vi "fit_fix height and width.vi"() -> ()   [LabVIEW 2016] (continued)
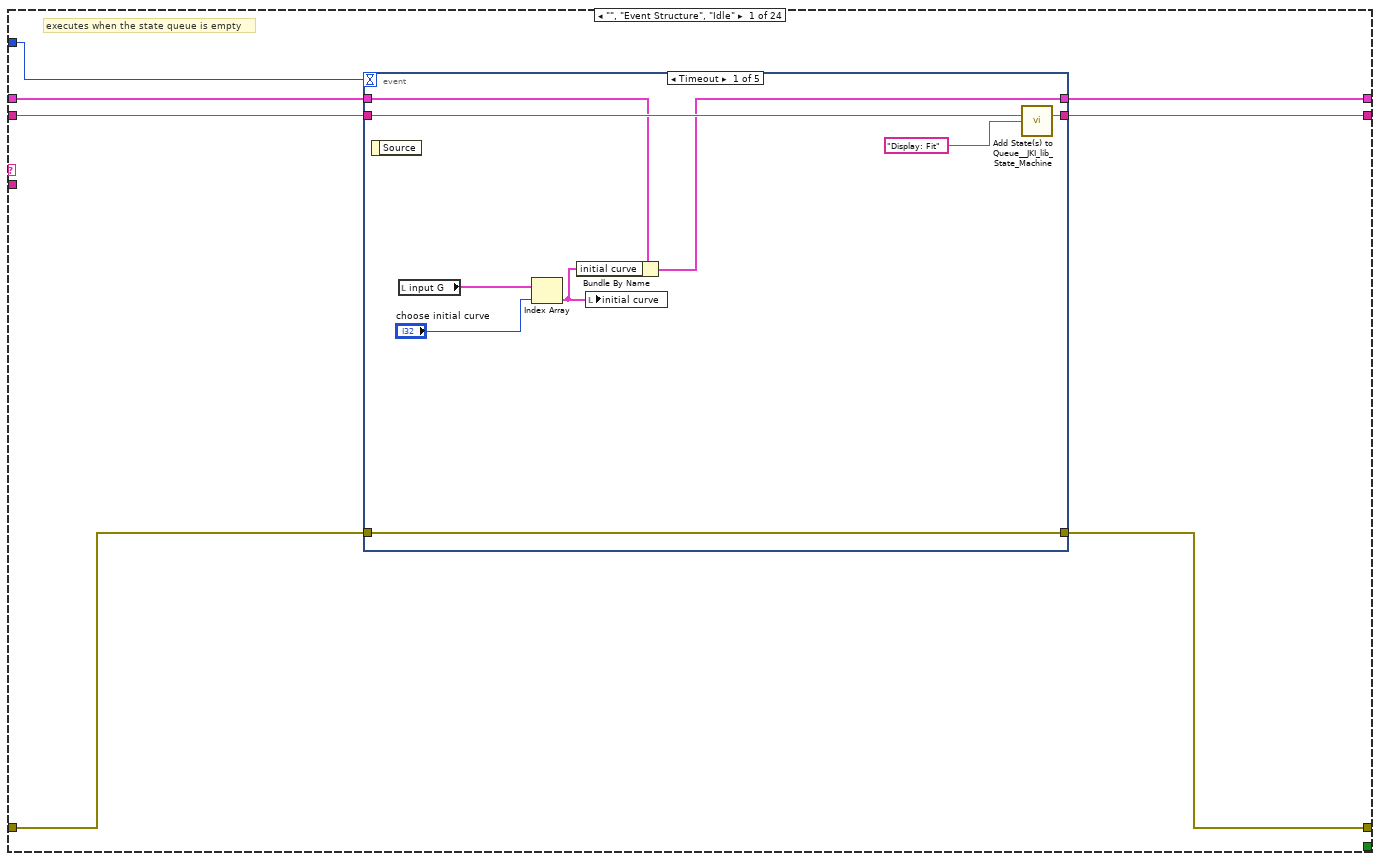
[diagram p3: hidden frame]
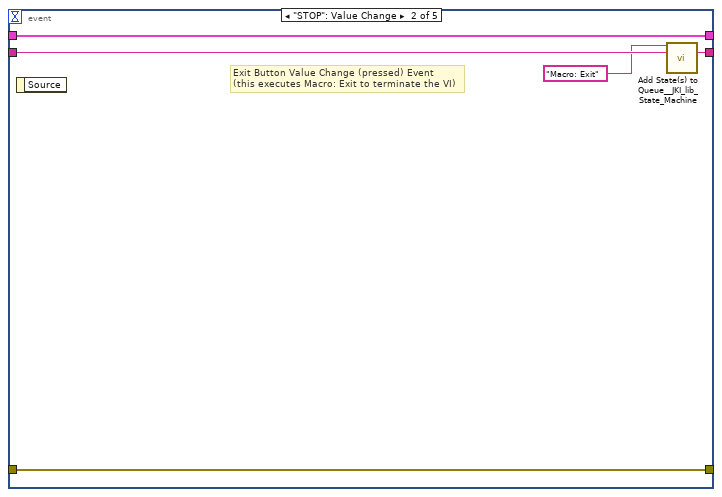
[diagram p4: hidden frame]
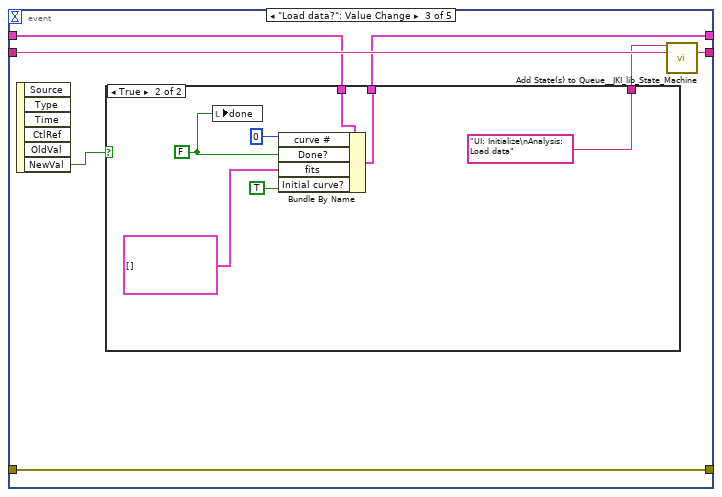
[diagram p5: hidden frame]
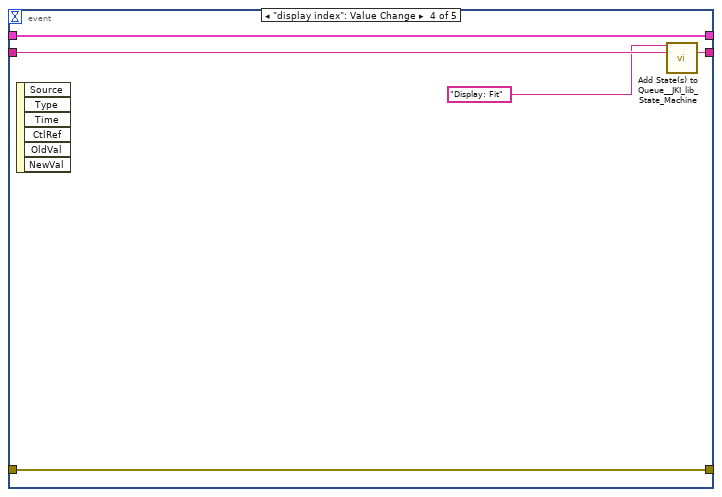
[diagram p7: hidden frame]
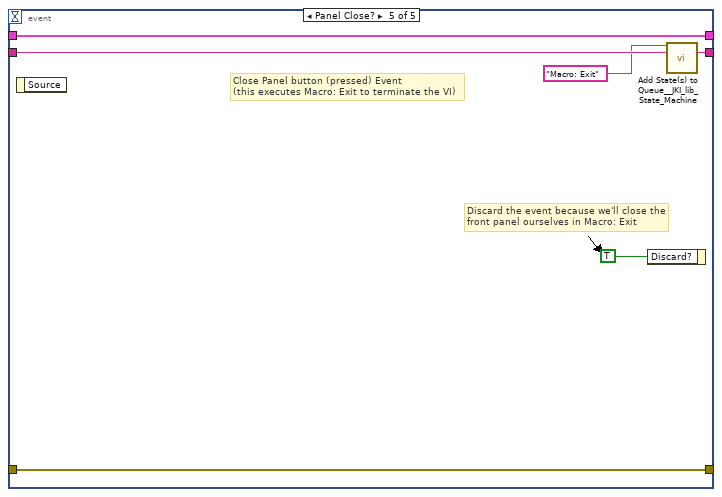
[diagram p8: hidden frame]
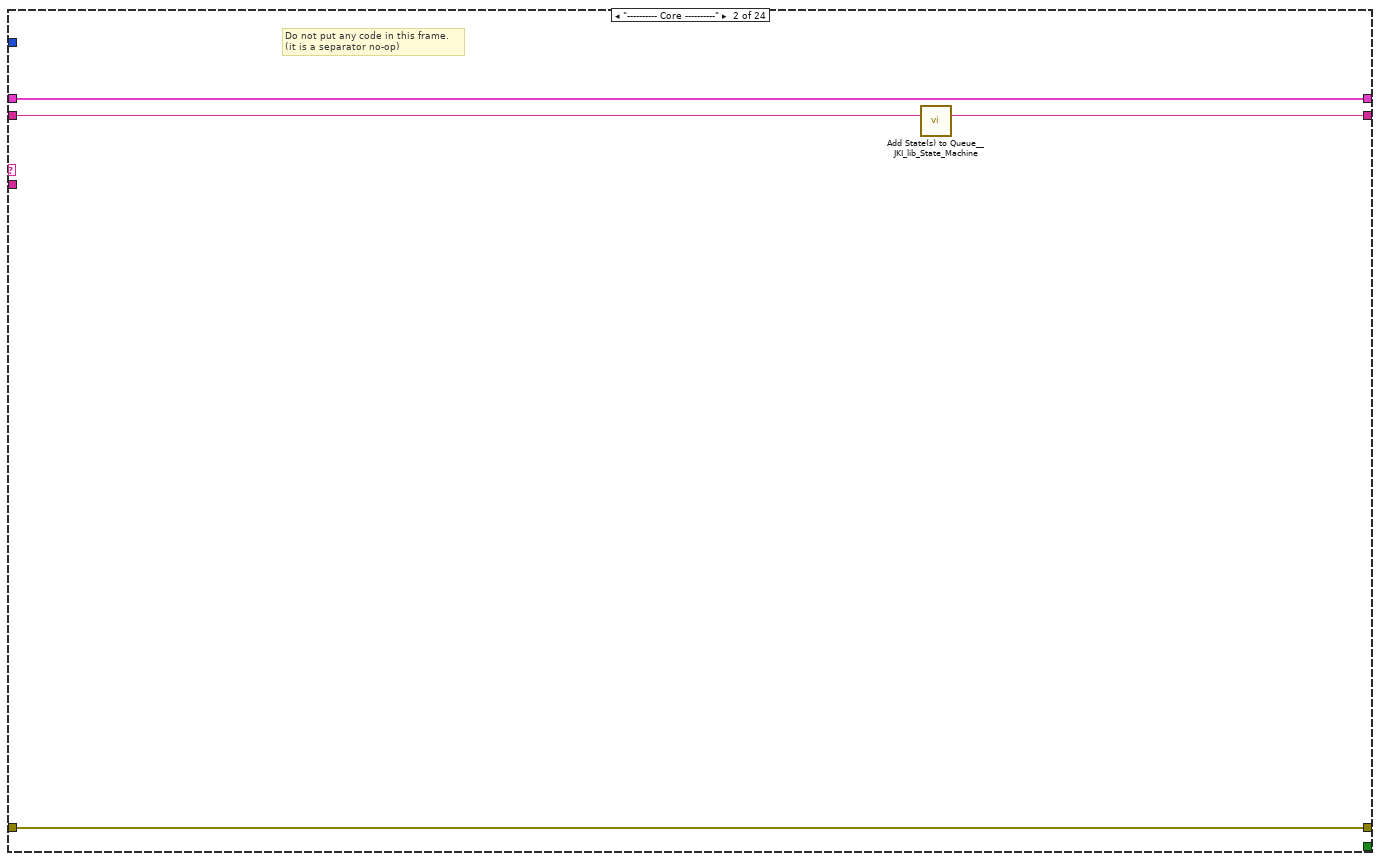
[diagram p9: hidden frame]
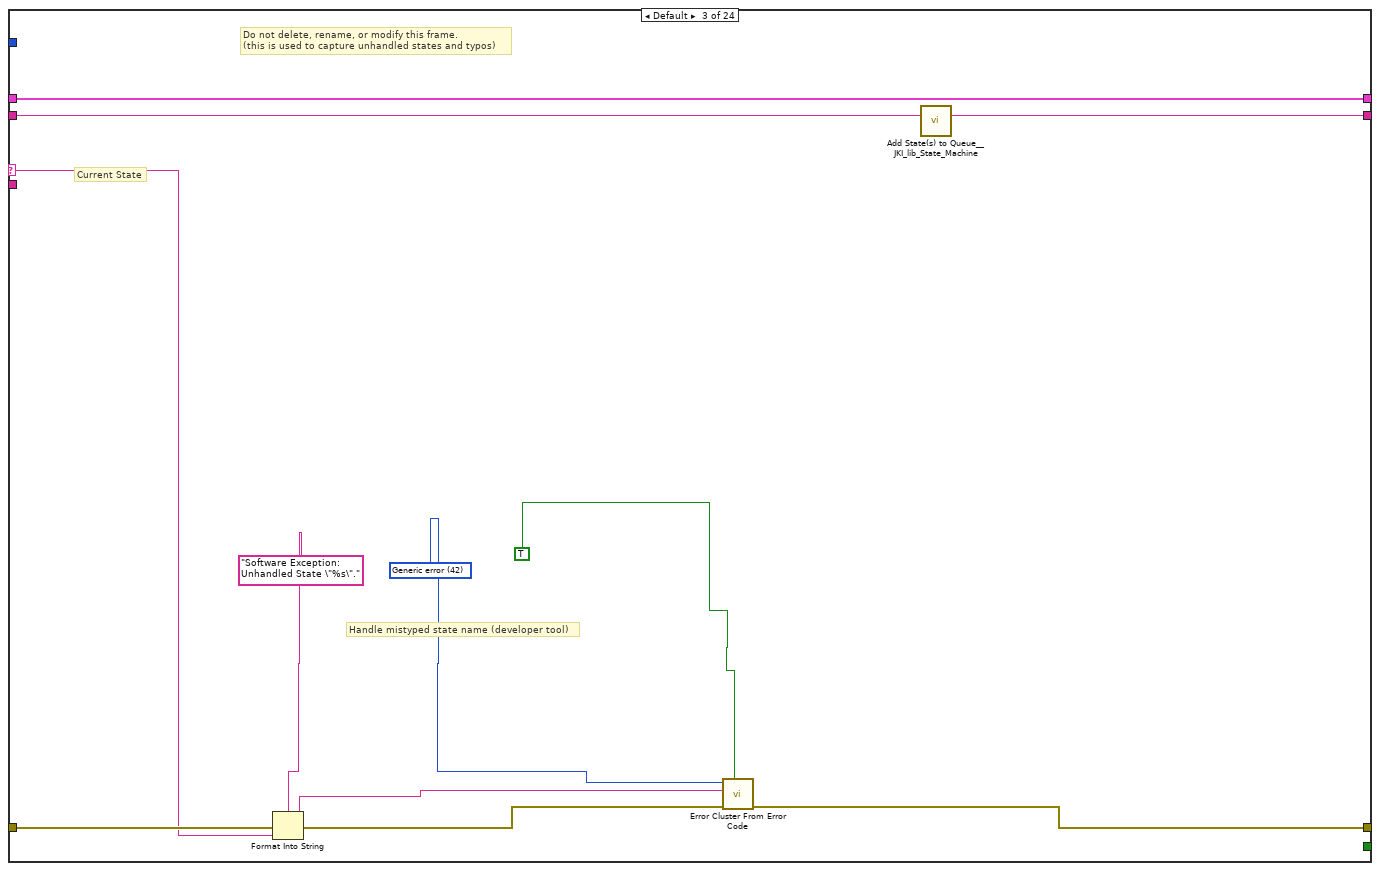
[diagram p10: hidden frame]
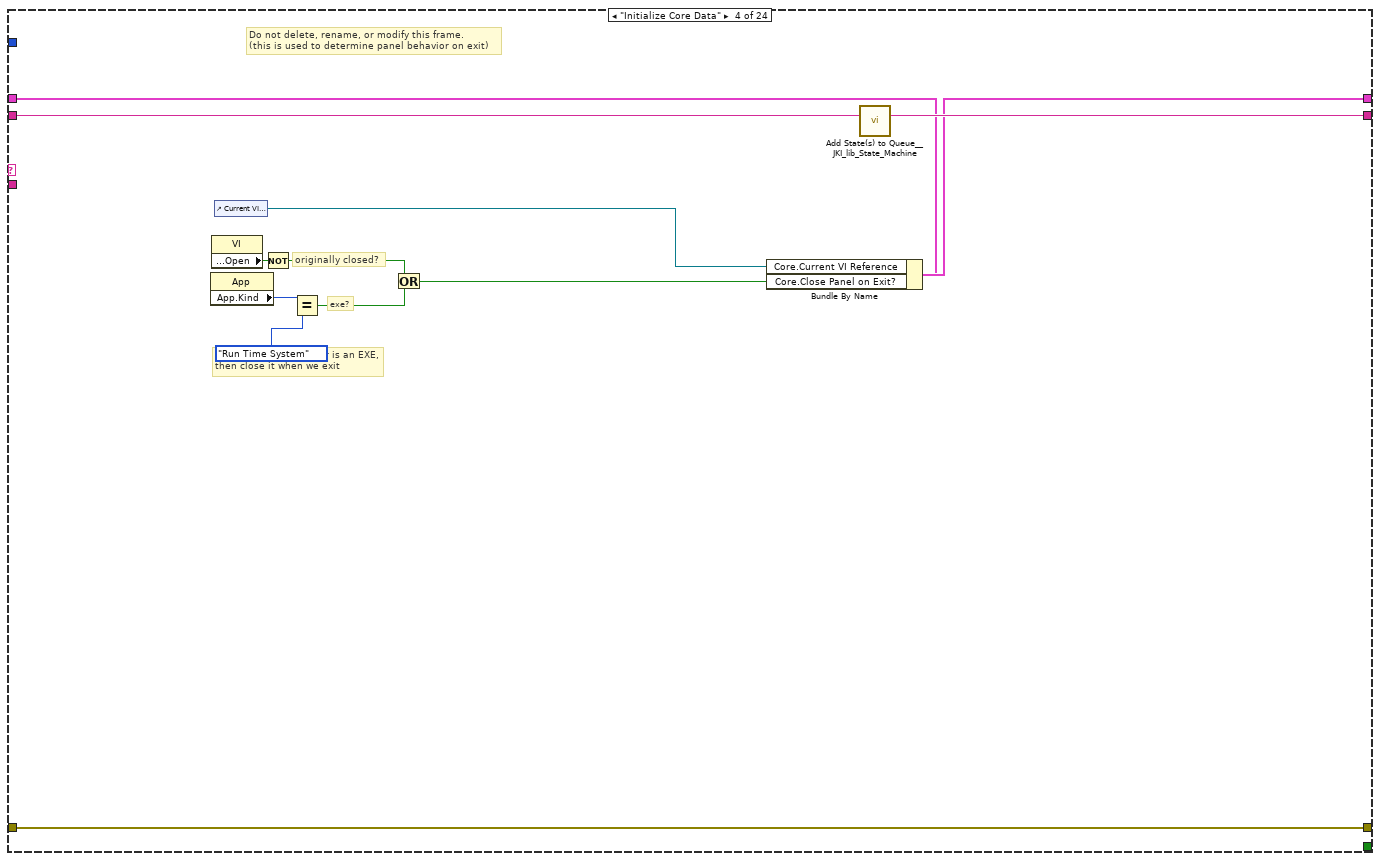
[diagram p11: hidden frame]
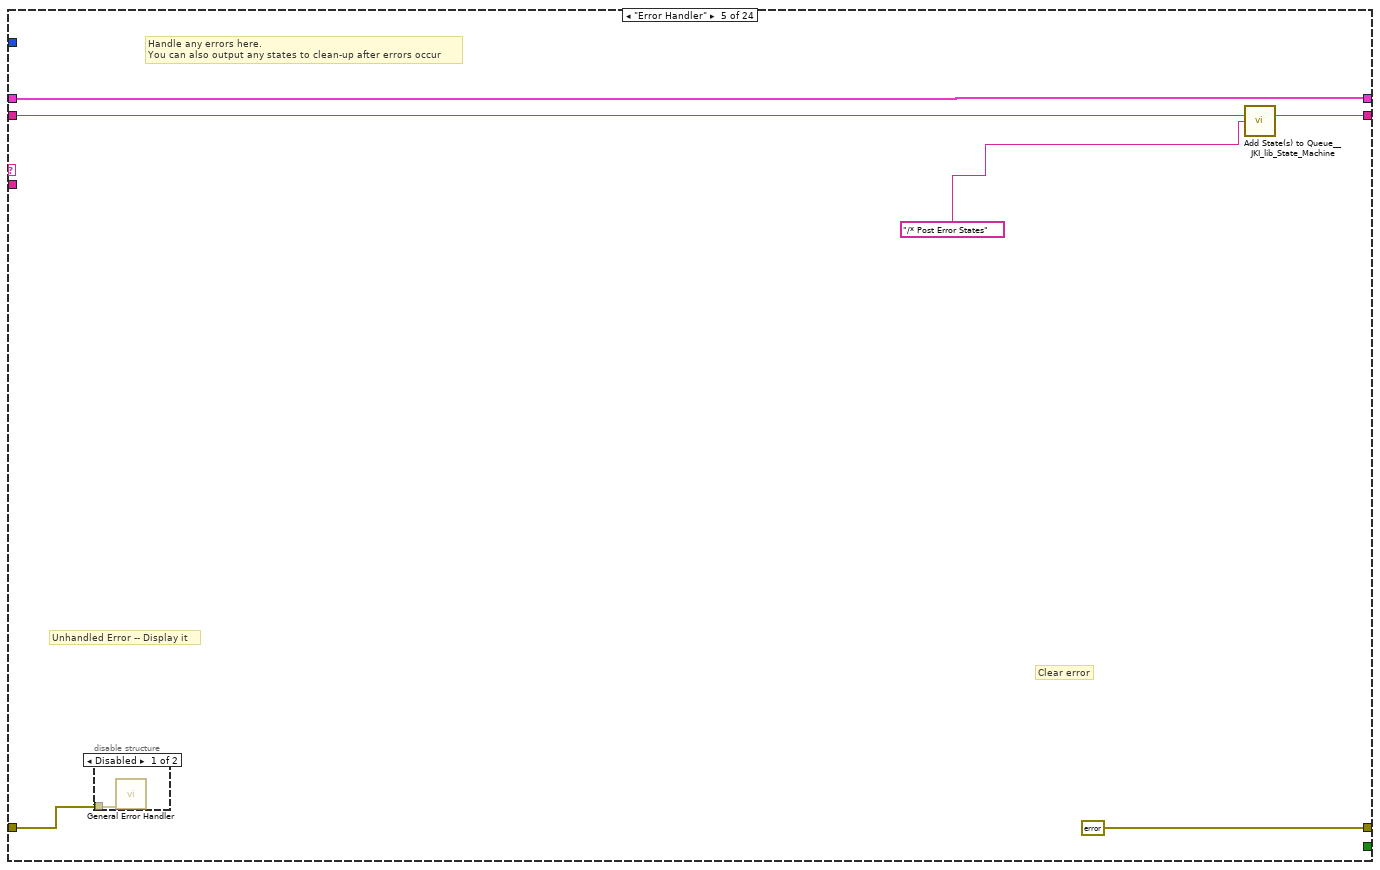
[diagram p12: hidden frame]
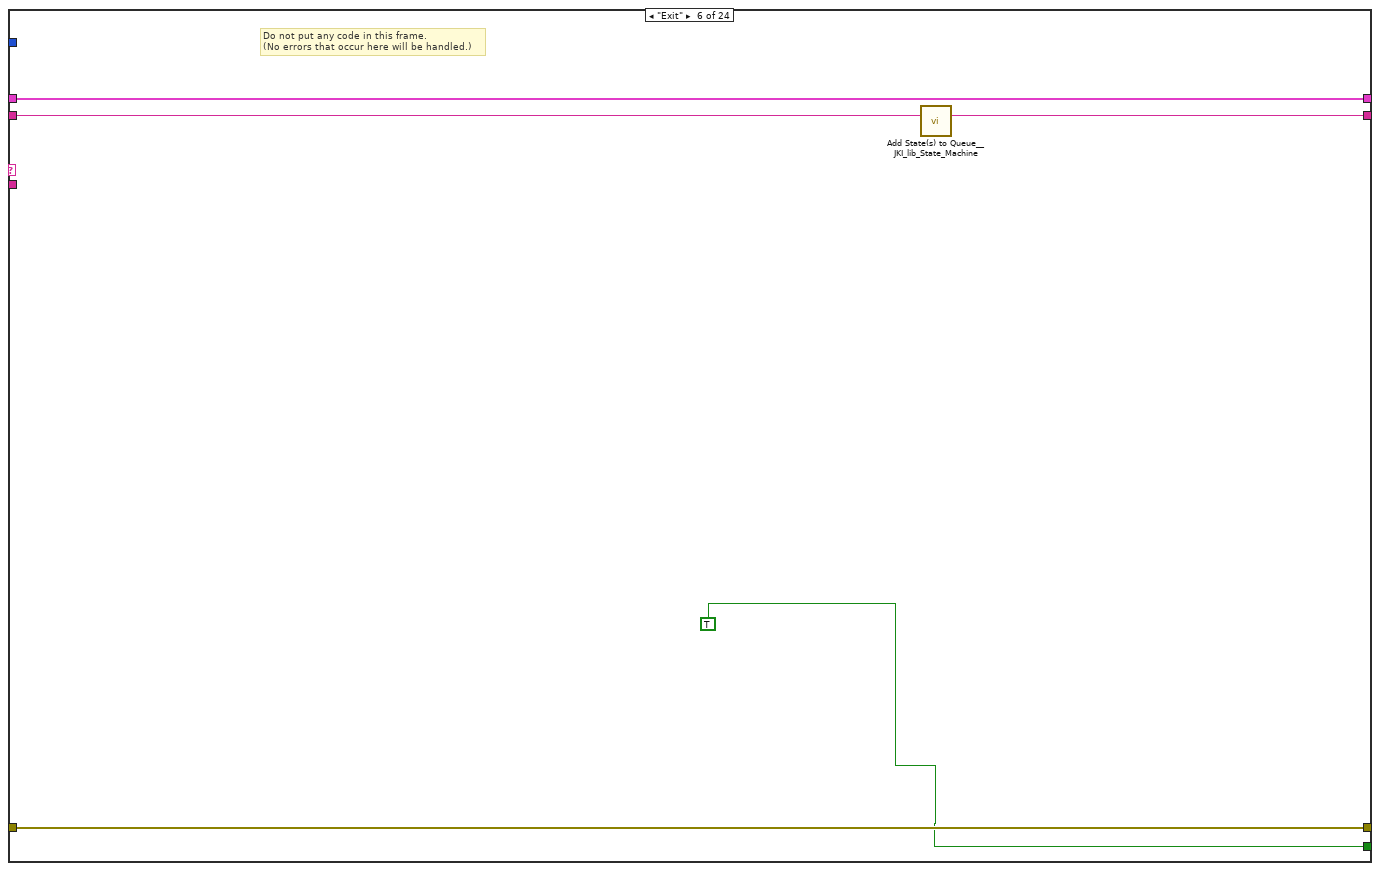
[diagram p14: hidden frame]
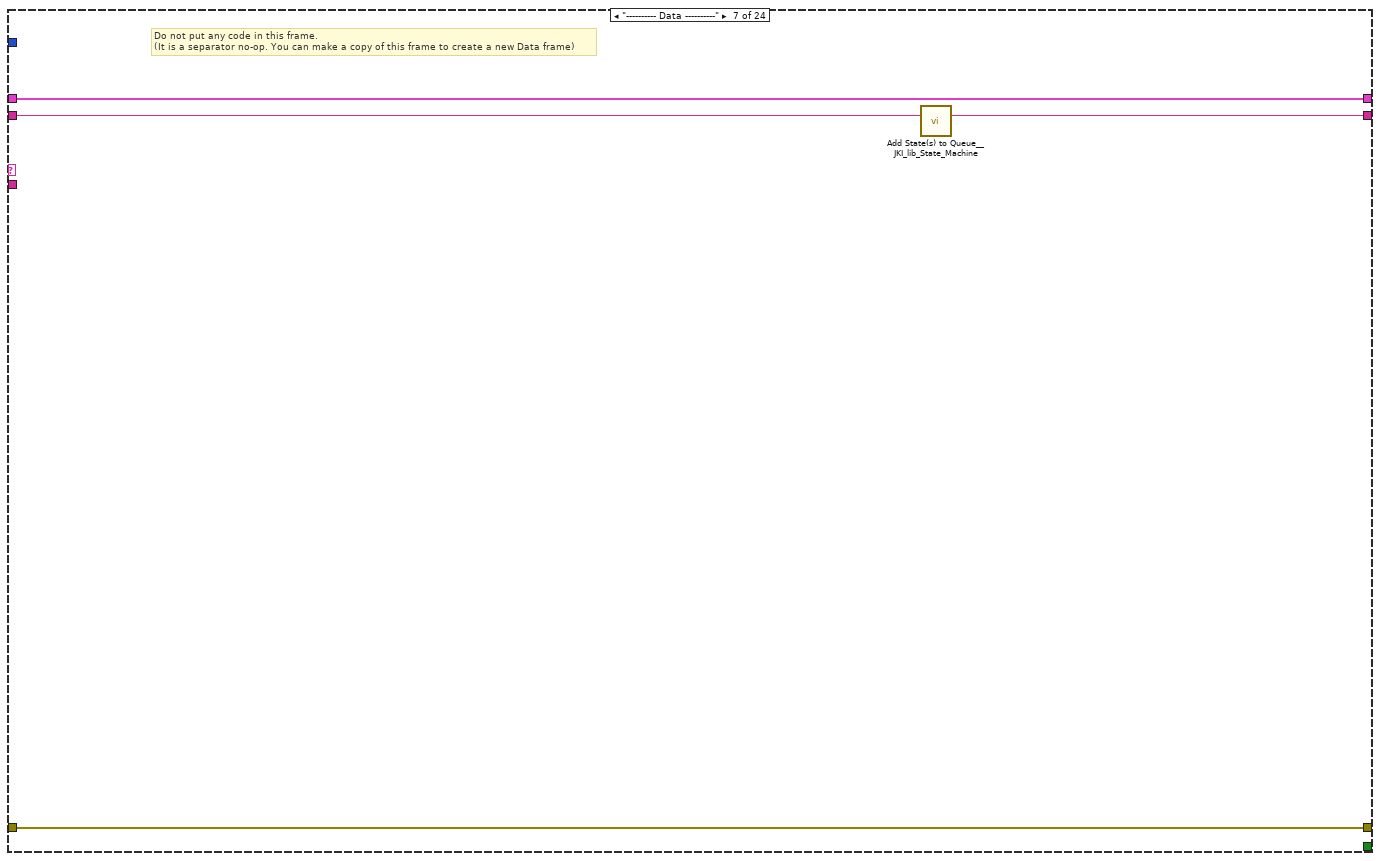
[diagram p15: hidden frame]
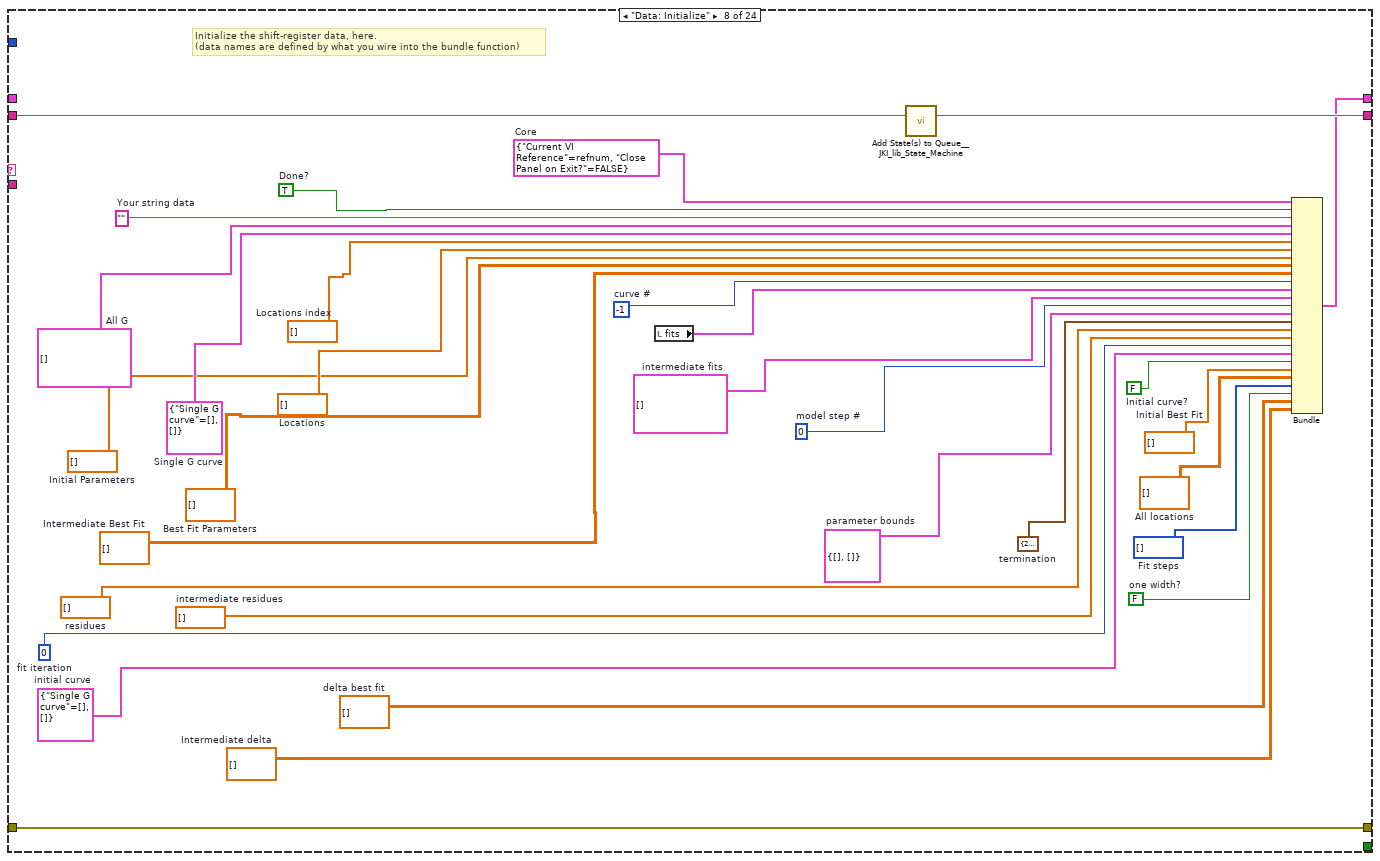
[diagram p16: hidden frame]
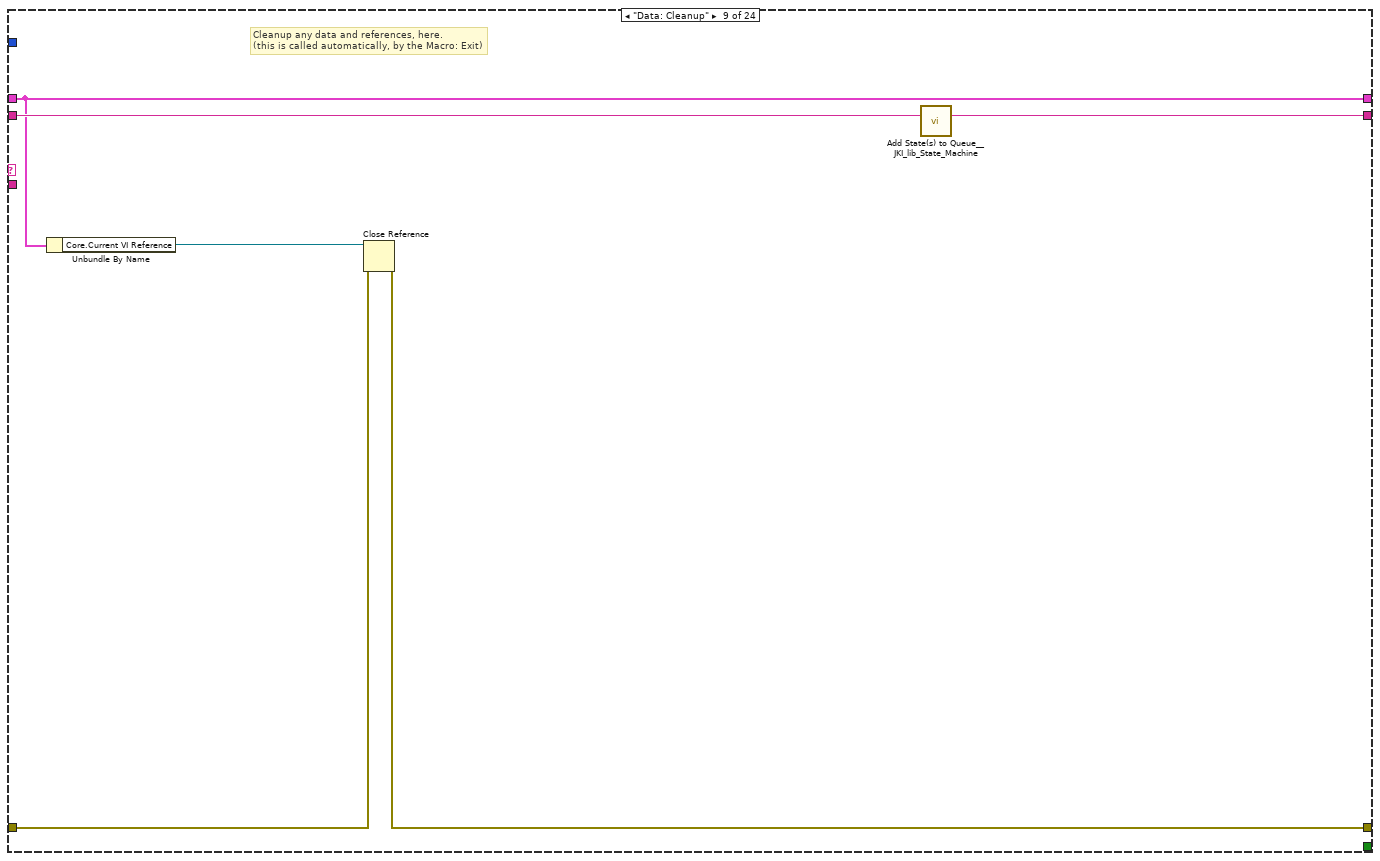
[diagram p17: hidden frame]
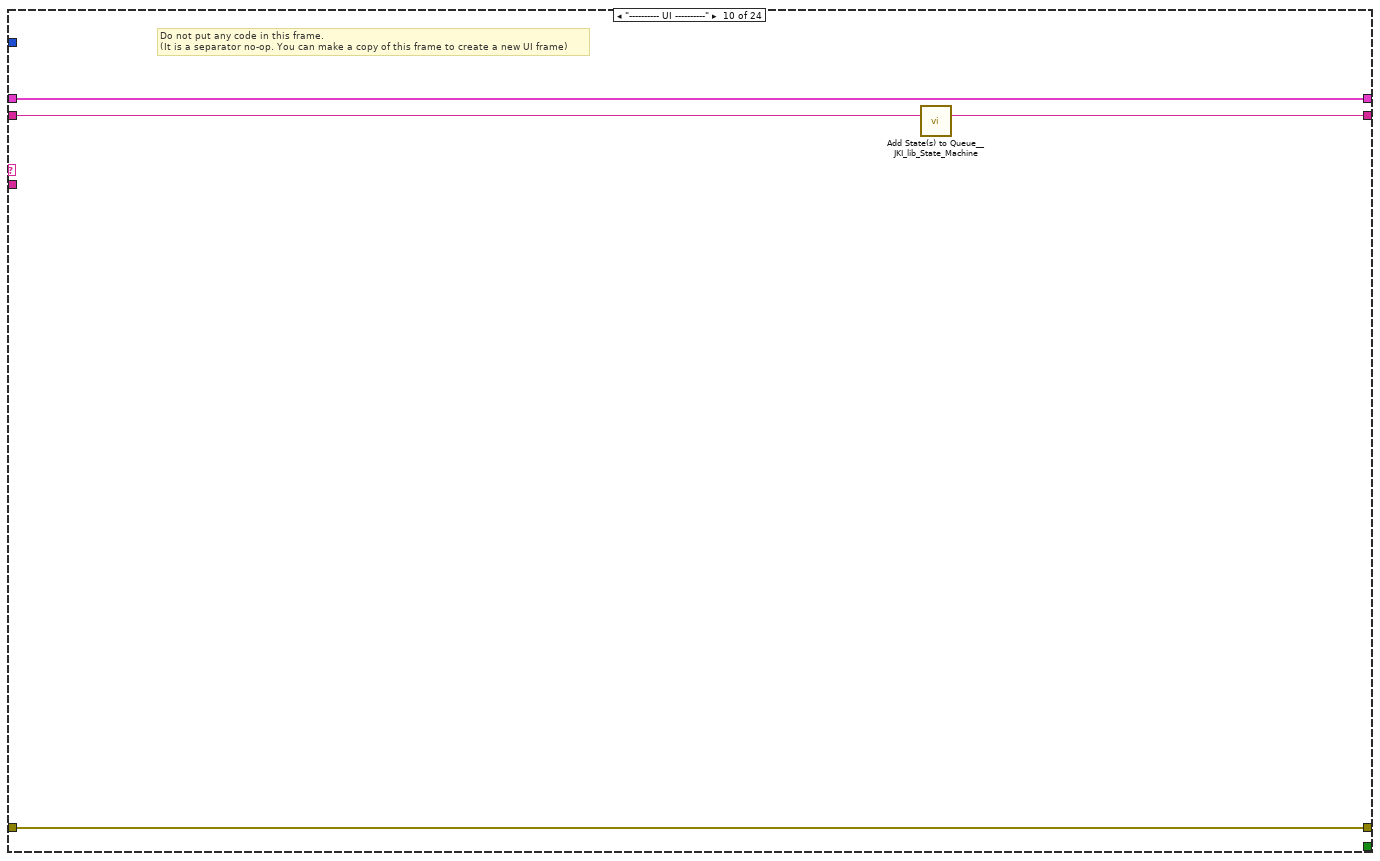
[diagram p18: hidden frame]
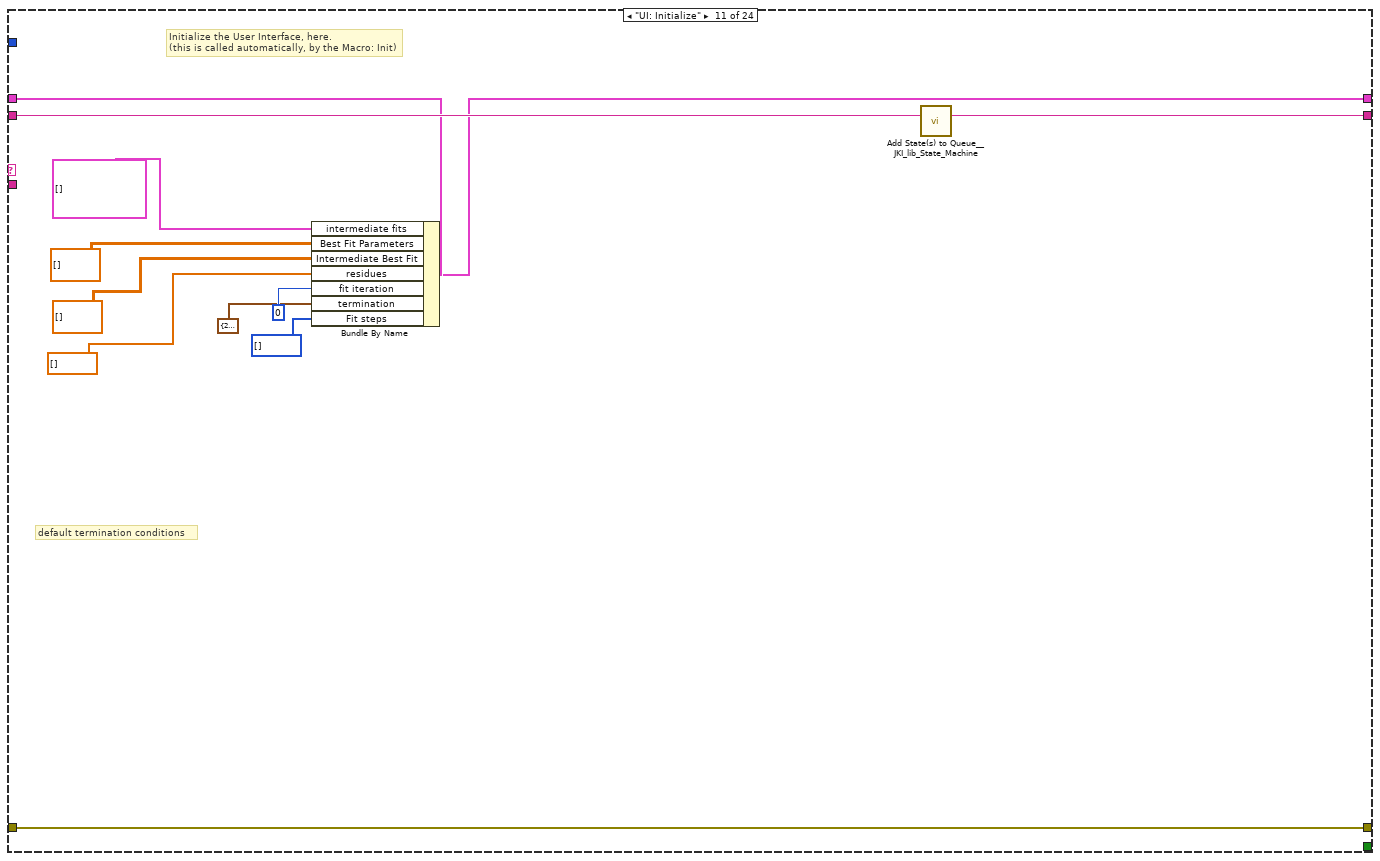
[diagram p19: hidden frame]
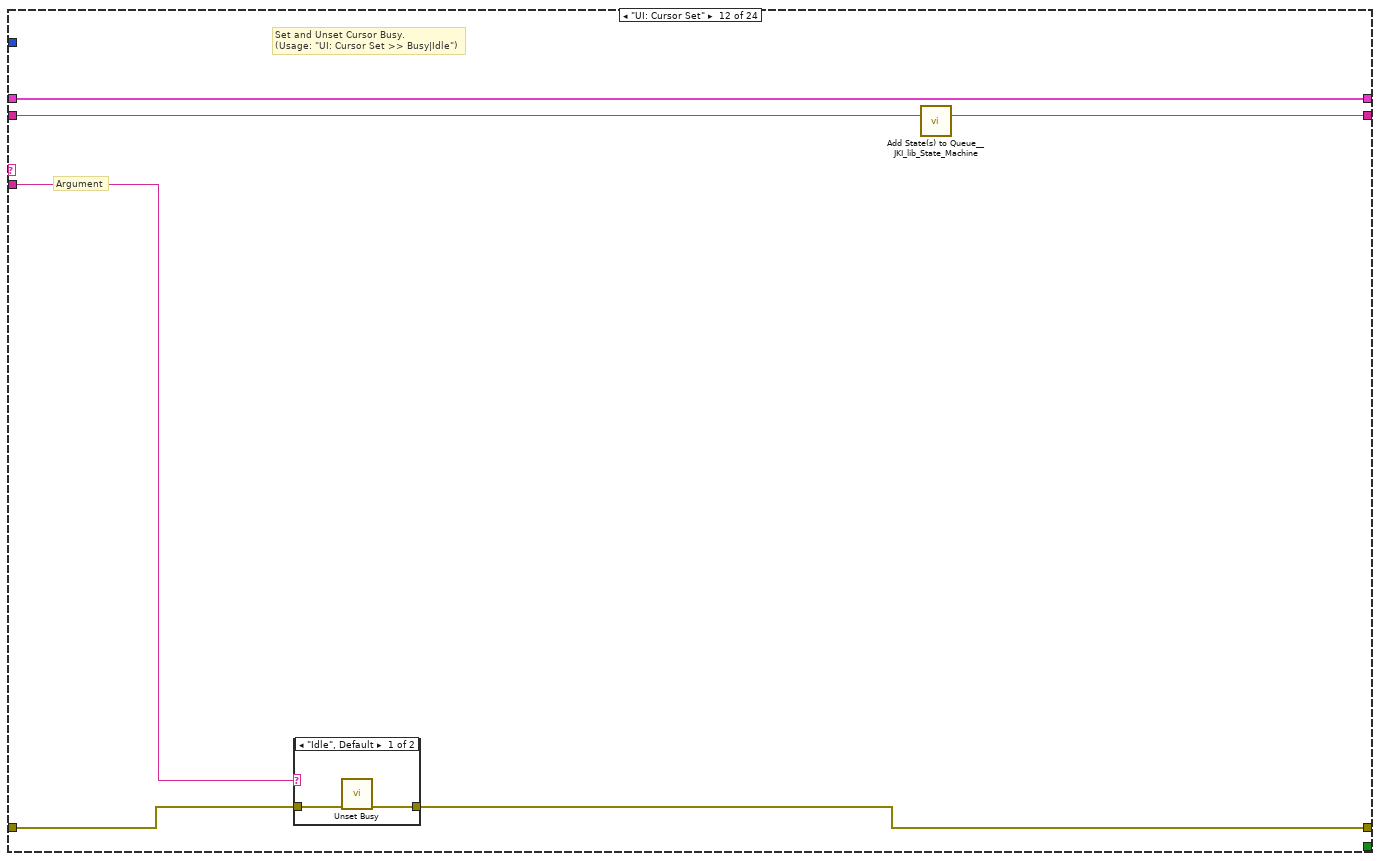
[diagram p20: hidden frame]
              n254 = call-poly <userlib>:"Reorder Array2__ogtk.vi"("indices"=w767, "array"=w776) -> ("reordered array"=w774:dbl[])  [unwired: 9 in]
              n255 = call-poly <userlib>:"Reorder Array2__ogtk.vi"("indices"=w767, "array"=w769) -> ()  [unwired: 9 in, 1 out]
              n256 = call-poly <userlib>:"Reorder Array2__ogtk.vi"("indices"=w767, "array"=w768) -> ("reordered array"=w766:dbl[])  [unwired: 9 in]
            }
          }
        }
        n257 = Index Array(array=w714, index (row)="display index") -> (element=→"Display best fit parameters":dbl[])  [unwired: 1 in]
        n258 = local write "fits"(w716) -> ()
        n259 = for {
          N: w712 -> [_]
          tunnel: w667 -> [w814]
          tunnel: [w821] -> w685 mode=indexing
          tunnel: w715 -> [w819]
          tunnel: w681 -> [w818]
          tunnel: [w816] -> w680 mode=indexing
          tunnel: w679 -> [w815]
          tunnel: [w812] -> w678 mode=indexing
          tunnel: w668 -> [w811]
          tunnel: w667 -> [w809]
          tunnel: [w807] -> w666 mode=indexing
          i -> [w810]
          n260 = Index Array(array=w811, index (col)=w810) -> (element=w808:dbl[])  [unwired: 1 in]
          n261 = Index Array(array=w819, index (col)=w810) -> (element=w820:dbl[])  [unwired: 1 in]
          n262 = Index Array(array=w818, index (col)=w810) -> (element=w817:dbl[])  [unwired: 1 in]
          n263 = Index Array(array=w815, index (col)=w810) -> (element=w813:dbl[])  [unwired: 1 in]
          n264 = Bundle(w814, "Sorted Array out"=w820) -> (w821:cluster{dbl[], "Sorted Array out":dbl[]})  [unwired: 1 in]
          n265 = Bundle(w814, "reordered array"=w817) -> (w816:cluster{dbl[], "reordered array":dbl[]})  [unwired: 1 in]
          n266 = Bundle(w809, "reordered array"=w808) -> (w807:cluster{dbl[], "reordered array":dbl[]})  [unwired: 1 in]
          n267 = Bundle(w814, "Best Fit Parameters"=w813) -> (w812:cluster{dbl[], "Best Fit Parameters":dbl[]})  [unwired: 1 in]
        }
        "amplitudes" <- w680
        "widths" <- w678
        "position errors" <- w666
        n268 = local write "Restricted G"(w721) -> ()
        n269 = Index Array(array=w721, index="display index") -> (element=w677:cluster{dbl[], dbl[]})
        n270 = Index Array(array=w716, index="display index") -> (element=w676:cluster{dbl[], dbl[]})
        n271 = Unbundle(w677) -> (w673:dbl[], w675:dbl[])
        n272 = Unbundle(w676) -> (w674:dbl[])  [unwired: 1 out]
        n273 = Subtract(x=w675, y=w674) -> (x-y=w672:dbl[])
        n274 = call <vilib>:"Add State(s) to Queue__JKI_lib_State_Machine.vi"("State(s) in (\"\")"=w726) -> ("States Out"=w725:string)  [unwired: 14 in]
        n275 = local write "fits 2"(w685) -> ()
        n276 = Bundle(w673, w672) -> (w671:cluster{dbl[], dbl[]})  [unwired: 1 in]
        n277 = Index Array(array=w685, index #1="pair index 1", index #2="pair index 2") -> (element #1=w709:cluster{dbl[], "Sorted Array out":dbl[]}, element #2=w708:cluster{dbl[], "Sorted Array out":dbl[]})
        n278 = Index Array(array=w685, index #1="trion index 1", index #2="trion index 2", index #3="trion index 3") -> (element #1=w701:cluster{dbl[], "Sorted Array out":dbl[]}, element #2=w700:cluster{dbl[], "Sorted Array out":dbl[]}, element #3=w699:cluster{dbl[], "Sorted Array out":dbl[]})
        n279 = Unbundle(w709) -> (w706:dbl[], "Sorted Array out"=w684:dbl[])
        n280 = Unbundle(w708) -> ("Sorted Array out"=w683:dbl[])  [unwired: 1 out]
        n281 = Unbundle(w699) -> ("Sorted Array out"=w692:dbl[])  [unwired: 1 out]
        n282 = Unbundle(w700) -> ("Sorted Array out"=w693:dbl[])  [unwired: 1 out]
        n283 = Unbundle(w701) -> (w691:dbl[], "Sorted Array out"=w694:dbl[])
        n284 = Build Array(w677, w676, w671) -> (w722:cluster{dbl[], dbl[]}[])
        n285 = for {
          tunnel: w694 -> [w801] mode=indexing
          tunnel: w693 -> [w800] mode=indexing
          tunnel: w692 -> [w799] mode=indexing
          tunnel: [w797] -> w689 mode=indexing
          n286 = Build Array(w801, w800, w799) -> (w798:dbl[])
          n287 = call <vilib>:"Std Deviation and Variance.vi"("X"=w798) -> ("standard deviation"=w797:dbl)  [unwired: 1 in, 2 out]
        }
        n288 = for {
          tunnel: w684 -> [w796] mode=indexing
          tunnel: w683 -> [w795] mode=indexing
          tunnel: [w793] -> w682 mode=indexing
          n289 = Build Array(w796, w795) -> (w794:dbl[])
          n290 = call <vilib>:"Std Deviation and Variance.vi"("X"=w794) -> ("standard deviation"=w793:dbl)  [unwired: 1 in, 2 out]
        }
        n291 = local write "display fit"(w722) -> ()
        n292 = Array Subset(array=w706, index="display index", length="display length") -> (w696:dbl[])
        n293 = Array Subset(array=w682, index="display index", length="display length") -> (w705:dbl[])
        n294 = Bundle(w696, w705) -> (→"pair":cluster{dbl[], dbl[]})  [unwired: 1 in]
        n295 = Array Subset(array=w691, index="display index 2", length="display length 2") -> (w690:dbl[])
        n296 = Array Subset(array=w689, index="display index 2", length="display length 2") -> (w688:dbl[])
        n297 = Bundle(w690, w688) -> (→"trion":cluster{dbl[], dbl[]})  [unwired: 1 in]
        "done" <- TRUE ("done")
      }
    }
  }
  n298 = disable-structure shown="Disabled" {
    frame Disabled {
      # "string model.vi ????"
      # "fitting sanity check"
      n299 = Unbundle() -> (w830)  [unwired: 1 in, 1 out]
      n300 = Concatenate Strings("y=" ("string"), ";" ("string")) -> (w828:string, w827:string)
      n301 = for {
        tunnel: _ -> [w841]
        tunnel: w830 -> [w842]
        tunnel: w828 -> [w839]
        tunnel: "x" ("x") -> [w838]
        tunnel: [w837] -> w824
        tunnel: string[] ["y"] ("Variables Output") -> [w835]
        tunnel: [w833] -> w829 mode=indexing
        tunnel: _ -> [w832]
        tunnel: [w831] -> _
        n302 = Build Array (concatenate)(w838, w837) -> (w836:string[])
        n303 = Build Array (concatenate)(w842, w841) -> (w840:void[])
        n304 = call <vilib>:"Eval Formula Node.vi"("Variables Input"=w836, "Input Values"=w840, "Variables Output"=w835, "formula"=w839, "error in (no error)"=w832) -> ("Output Values"=w834:dbl[], "error out"=w831:errorcluster)
        n305 = Index Array(array=w834) -> (element=w833:dbl)  [unwired: 1 in]
      }
      n306 = Bundle(w830, w829) -> ()  [unwired: 1 in, 1 out]
    }
    frame Enabled {
    }
  }
